vi "String to Array.vi"(10 "Input String":string) -> (2 "String Array":string[](array[string]))   [LabVIEW 2013]
doc: "This sub-VI splits a multi-line input string into an array of single-line strings and returns the array"
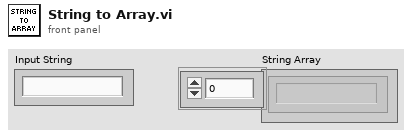
[diagram p1: front panel]
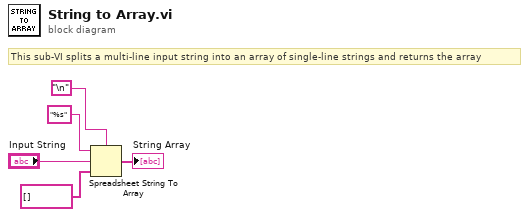
[diagram p0: block diagram]
diagram:
  # "This sub-VI splits a multi-line input string into an array of single-line strings and returns the array"
  n1 = Spreadsheet String To Array(delimiter (Tab)="\n", format string="%s", spreadsheet string="Input String", array type (2D Dbl)=string[] [] ("String Array 2")) -> (array=→"String Array":string[])
